vi "filter_param.vi"() -> (0 "shift 0.1":i32, 1 "shift 0.5":i32, 2 "Coeffs Fs=0.1":fxp<+/-,18,18>[](array[numeric]), 3 "Coeffs Fs=0.5":fxp<+/-,18,18>[](array[numeric]))   [LabVIEW 2013]
panel:
  out "sum 0.1":i32
  out "sum 0.5":i32
  out "Waveform Graph":i32[][](graph)
  out "subarray":string[](array[string])
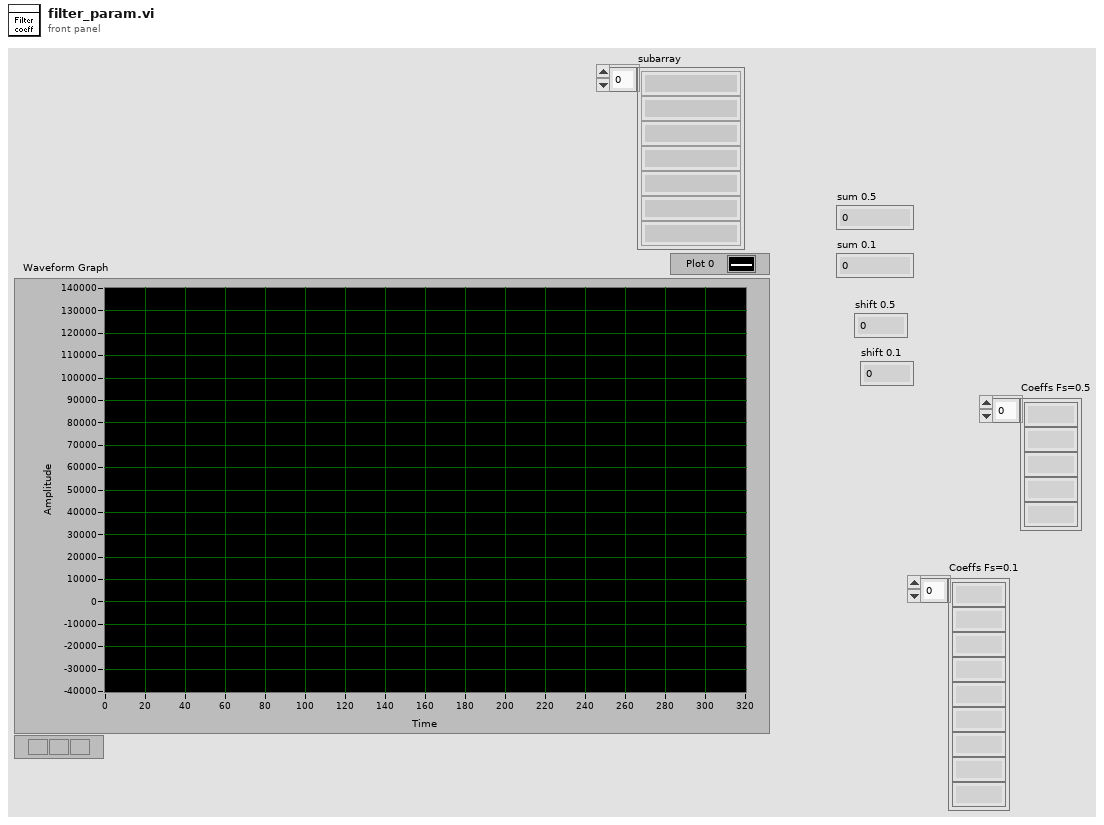
[diagram p1: front panel]
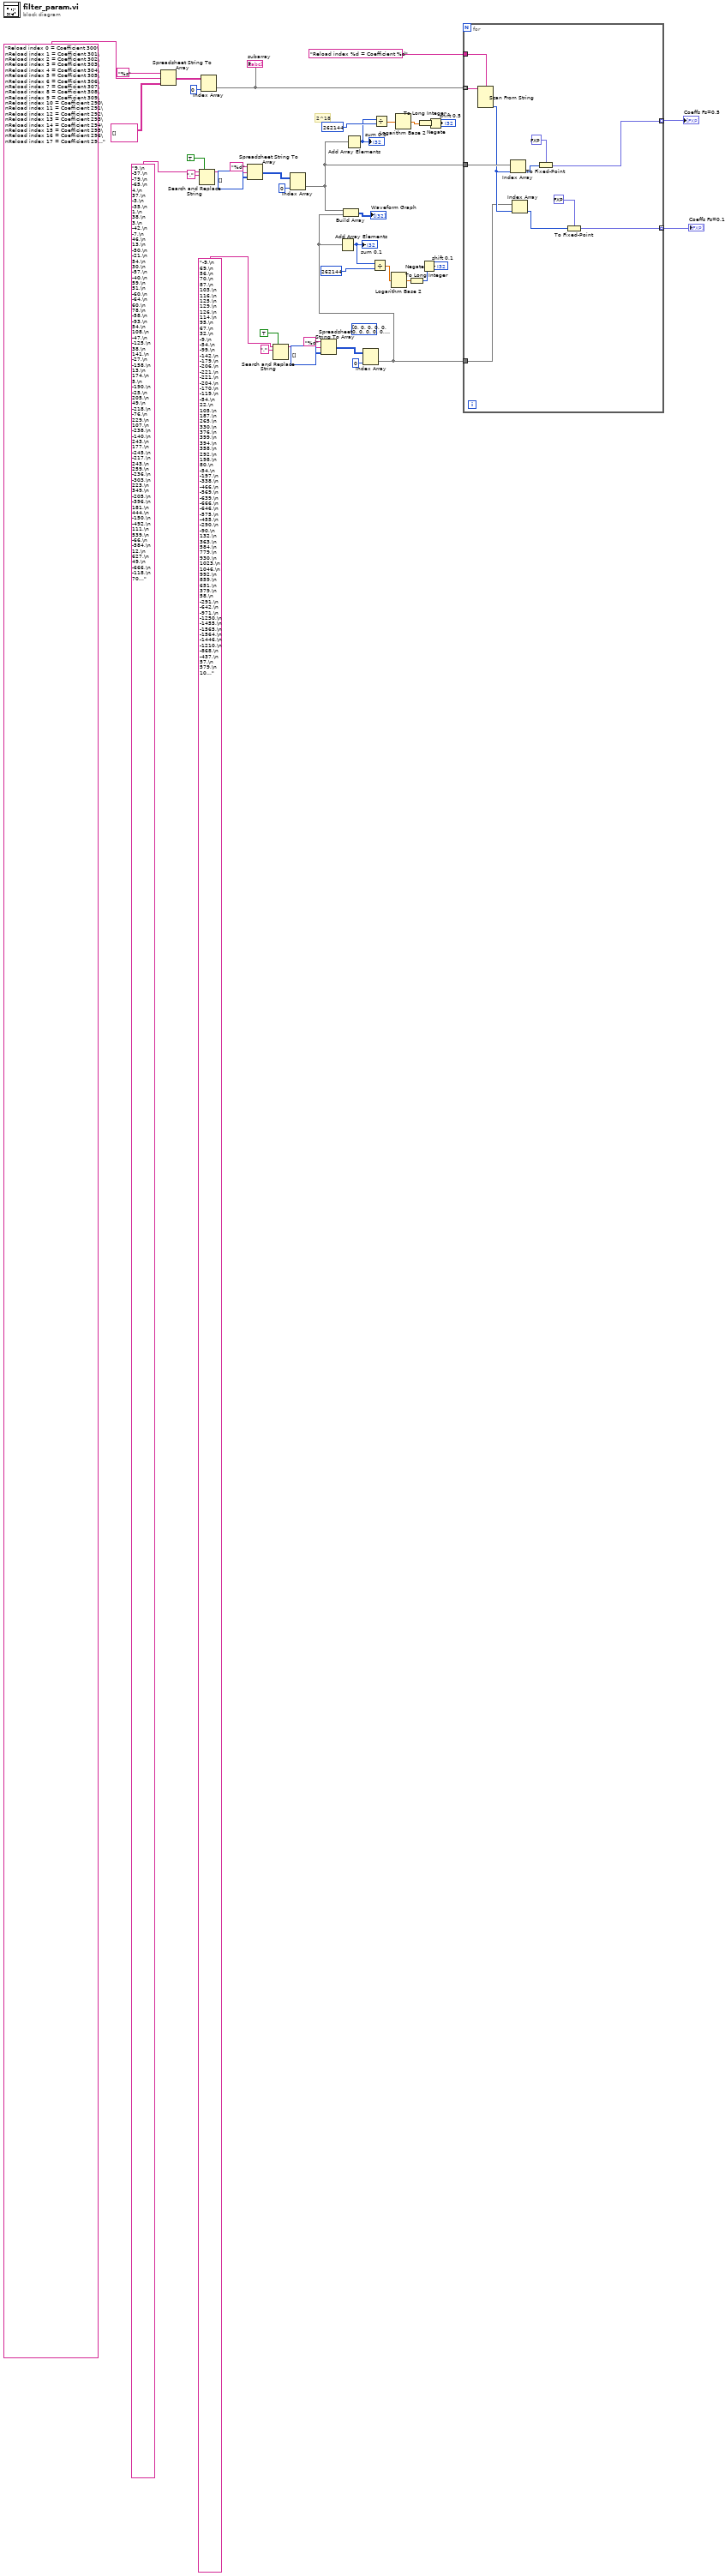
[diagram p0: block diagram]
diagram:
  (unwired) i32[] [0, 0, 0, 0, 0, 0, 0, 0, 0, 0, 0, 0, 0, 0, 0, 0, 0, 0, 0, 0, 0, 0, 0, 0, 0, 0, 0, 0, 0, 0, 0, 0, 0, 0, 0, 0, 0, 0, 0, 0, 0, 0, 0, 0, 0, 0, 0, 0, 0, 0, 0, 0, 0, 0, 0, 0, 0, 0, 0, 0, 0, 0, 0, 0, 0, 0, 0, 0, 0, 0, 0, 0, 0, 0, 0, 0, 0, 0, 0, 0, 0, 0, 0, 0, 0, 0, 0, 0, 0, 0, 0, 0, 0, 0, 0, 0, 0, 0, 0, 0, 0, 0, 0, 0, 0, 0, 0, 0, 0, 0, 0, 0, 0, 0, 0, 0, 0, 0, 0, 0, 0, 0, 0, 0, 0, 0, 0, 0, 0, 0, 0, -22, -91, -234, -449, -668, -741, -465, 327, 1628, 3128, 4186, 3968, 1771, -2547, -8192, -13332, -15398, -11800, -870, 17293, 40433, 64437, 84313, 95575, 95575, 84313, 64437, 40433, 17293, -870, -11800, -15398, -13332, -8192, -2547, 1771, 3968, 4186, 3128, 1628, 327, -465, -741, -668, -449, -234, -91, -22, 0, 0, 0, 0, 0, 0, 0, 0, 0, 0, 0, 0, 0, 0, 0, 0, 0, 0, 0, 0, 0, 0, 0, 0, 0, 0, 0, 0, 0, 0, 0, 0, 0, 0, 0, 0, 0, 0, 0, 0, 0, 0, 0, 0, 0, 0, 0, 0, 0, 0, 0, 0, 0, 0, 0, 0, 0, 0, 0, 0, 0, 0, 0, 0, 0, 0, 0, 0, 0, 0, 0, 0, 0, 0, 0, 0, 0, 0, 0, 0, 0, 0, 0, 0, 0, 0, 0, 0, 0, 0, 0, 0, 0, 0, 0, 0, 0, 0, 0, 0, 0, 0, 0, 0, 0, 0, 0, 0, 0, 0, 0, 0, 0, 0, 0, 0, 0, 0, 0, 0, 0, 0, 0, 0, 0, 0, 0, 0, 0, 0, 0] ("output array")
  # "2^18"
  n1 = Spreadsheet String To Array(format string="%s", spreadsheet string="Reload index 0 = Coefficient 300\nReload index 1 = Coefficient 301\nReload index 2 = Coefficient 302\nReload index 3 = Coefficient 303\nReload index 4 = Coefficient 304\nReload index 5 = Coefficient 305\nReload index 6 = Coefficient 306\nReload index 7 = Coefficient 307\nReload index 8 = Coefficient 308\nReload index 9 = Coefficient 309\nReload index 10 = Coefficient 290\nReload index 11 = Coefficient 291\nReload index 12 = Coefficient 292\nReload index 13 = Coefficient 293\nReload index 14 = Coefficient 294\nReload index 15 = Coefficient 295\nReload index 16 = Coefficient 296\nReload index 17 = Coefficient 297\nReload index 18 = Coefficient 298\nReload index 19 = Coefficient 299\nReload index 20 = Coefficient 280\nReload index 21 = Coefficient 281\nReload index 22 = Coefficient 282\nReload index 23 = Coefficient 283\nReload index 24 = Coefficient 284\nReload index 25 = Coefficient 285\nReload index 26 = Coefficient 286\nReload index 27 = Coefficient 287\nReload index 28 = Coefficient 288\nReload index 29 = Coefficient 289\nReload index 30 = Coefficient 270\nReload index 31 = Coefficient 271\nReload index 32 = Coefficient 272\nReload index 33 = Coefficient 273\nReload index 34 = Coefficient 274\nReload index 35 = Coefficient 275\nReload index 36 = Coefficient 276\nReload index 37 = Coefficient 277\nReload index 38 = Coefficient 278\nReload index 39 = Coefficient 279\nReload index 40 = Coefficient 260\nReload index 41 = Coefficient 261\nReload index 42 = Coefficient 262\nReload index 43 = Coefficient 263\nReload index 44 = Coefficient 264\nReload index 45 = Coefficient 265\nReload index 46 = Coefficient 266\nReload index 47 = Coefficient 267\nReload index 48 = Coefficient 268\nReload index 49 = Coefficient 269\nReload index 50 = Coefficient 250\nReload index 51 = Coefficient 251\nReload index 52 = Coefficient 252\nReload index 53 = Coefficient 253\nReload index 54 = Coefficient 254\nReload index 55 = Coefficient 255\nReload index 56 = Coefficient 256\nReload index 57 = Coefficient 257\nReload index 58 = Coefficient 258\nReload index 59 = Coefficient 259\nReload index 60 = Coefficient 240\nReload index 61 = Coefficient 241\nReload index 62 = Coefficient 242\nReload index 63 = Coefficient 243\nReload index 64 = Coefficient 244\nReload index 65 = Coefficient 245\nReload index 66 = Coefficient 246\nReload index 67 = Coefficient 247\nReload index 68 = Coefficient 248\nReload index 69 = Coefficient 249\nReload index 70 = Coefficient 230\nReload index 71 = Coefficient 231\nReload index 72 = Coefficient 232\nReload index 73 = Coefficient 233\nReload index 74 = Coefficient 234\nReload index 75 = Coefficient 235\nReload index 76 = Coefficient 236\nReload index 77 = Coefficient 237\nReload index 78 = Coefficient 238\nReload index 79 = Coefficient 239\nReload index 80 = Coefficient 220\nReload index 81 = Coefficient 221\nReload index 82 = Coefficient 222\nReload index 83 = Coefficient 223\nReload index 84 = Coefficient 224\nReload index 85 = Coefficient 225\nReload index 86 = Coefficient 226\nReload index 87 = Coefficient 227\nReload index 88 = Coefficient 228\nReload index 89 = Coefficient 229\nReload index 90 = Coefficient 210\nReload index 91 = Coefficient 211\nReload index 92 = Coefficient 212\nReload index 93 = Coefficient 213\nReload index 94 = Coefficient 214\nReload index 95 = Coefficient 215\nReload index 96 = Coefficient 216\nReload index 97 = Coefficient 217\nReload index 98 = Coefficient 218\nReload index 99 = Coefficient 219\nReload index 100 = Coefficient 200\nReload index 101 = Coefficient 201\nReload index 102 = Coefficient 202\nReload index 103 = Coefficient 203\nReload index 104 = Coefficient 204\nReload index 105 = Coefficient 205\nReload index 106 = Coefficient 206\nReload index 107 = Coefficient 207\nReload index 108 = Coefficient 208\nReload index 109 = Coefficient 209\nReload index 110 = Coefficient 190\nReload index 111 = Coefficient 191\nReload index 112 = Coefficient 192\nReload index 113 = Coefficient 193\nReload index 114 = Coefficient 194\nReload index 115 = Coefficient 195\nReload index 116 = Coefficient 196\nReload index 117 = Coefficient 197\nReload index 118 = Coefficient 198\nReload index 119 = Coefficient 199\nReload index 120 = Coefficient 180\nReload index 121 = Coefficient 181\nReload index 122 = Coefficient 182\nReload index 123 = Coefficient 183\nReload index 124 = Coefficient 184\nReload index 125 = Coefficient 185\nReload index 126 = Coefficient 186\nReload index 127 = Coefficient 187\nReload index 128 = Coefficient 188\nReload index 129 = Coefficient 189\nReload index 130 = Coefficient 170\nReload index 131 = Coefficient 171\nReload index 132 = Coefficient 172\nReload index 133 = Coefficient 173\nReload index 134 = Coefficient 174\nReload index 135 = Coefficient 175\nReload index 136 = Coefficient 176\nReload index 137 = Coefficient 177\nReload index 138 = Coefficient 178\nReload index 139 = Coefficient 179\nReload index 140 = Coefficient 160\nReload index 141 = Coefficient 161\nReload index 142 = Coefficient 162\nReload index 143 = Coefficient 163\nReload index 144 = Coefficient 164\nReload index 145 = Coefficient 165\nReload index 146 = Coefficient 166\nReload index 147 = Coefficient 167\nReload index 148 = Coefficient 168\nReload index 149 = Coefficient 169\nReload index 150 = Coefficient 150\nReload index 151 = Coefficient 151\nReload index 152 = Coefficient 152\nReload index 153 = Coefficient 153\nReload index 154 = Coefficient 154\nReload index 155 = Coefficient 155\nReload index 156 = Coefficient 156\nReload index 157 = Coefficient 157\nReload index 158 = Coefficient 158\nReload index 159 = Coefficient 159\nReload index 160 = Coefficient 140\nReload index 161 = Coefficient 141\nReload index 162 = Coefficient 142\nReload index 163 = Coefficient 143\nReload index 164 = Coefficient 144\nReload index 165 = Coefficient 145\nReload index 166 = Coefficient 146\nReload index 167 = Coefficient 147\nReload index 168 = Coefficient 148\nReload index 169 = Coefficient 149\nReload index 170 = Coefficient 130\nReload index 171 = Coefficient 131\nReload index 172 = Coefficient 132\nReload index 173 = Coefficient 133\nReload index 174 = Coefficient 134\nReload index 175 = Coefficient 135\nReload index 176 = Coefficient 136\nReload index 177 = Coefficient 137\nReload index 178 = Coefficient 138\nReload index 179 = Coefficient 139\nReload index 180 = Coefficient 120\nReload index 181 = Coefficient 121\nReload index 182 = Coefficient 122\nReload index 183 = Coefficient 123\nReload index 184 = Coefficient 124\nReload index 185 = Coefficient 125\nReload index 186 = Coefficient 126\nReload index 187 = Coefficient 127\nReload index 188 = Coefficient 128\nReload index 189 = Coefficient 129\nReload index 190 = Coefficient 110\nReload index 191 = Coefficient 111\nReload index 192 = Coefficient 112\nReload index 193 = Coefficient 113\nReload index 194 = Coefficient 114\nReload index 195 = Coefficient 115\nReload index 196 = Coefficient 116\nReload index 197 = Coefficient 117\nReload index 198 = Coefficient 118\nReload index 199 = Coefficient 119\nReload index 200 = Coefficient 100\nReload index 201 = Coefficient 101\nReload index 202 = Coefficient 102\nReload index 203 = Coefficient 103\nReload index 204 = Coefficient 104\nReload index 205 = Coefficient 105\nReload index 206 = Coefficient 106\nReload index 207 = Coefficient 107\nReload index 208 = Coefficient 108\nReload index 209 = Coefficient 109\nReload index 210 = Coefficient 90\nReload index 211 = Coefficient 91\nReload index 212 = Coefficient 92\nReload index 213 = Coefficient 93\nReload index 214 = Coefficient 94\nReload index 215 = Coefficient 95\nReload index 216 = Coefficient 96\nReload index 217 = Coefficient 97\nReload index 218 = Coefficient 98\nReload index 219 = Coefficient 99\nReload index 220 = Coefficient 80\nReload index 221 = Coefficient 81\nReload index 222 = Coefficient 82\nReload index 223 = Coefficient 83\nReload index 224 = Coefficient 84\nReload index 225 = Coefficient 85\nReload index 226 = Coefficient 86\nReload index 227 = Coefficient 87\nReload index 228 = Coefficient 88\nReload index 229 = Coefficient 89\nReload index 230 = Coefficient 70\nReload index 231 = Coefficient 71\nReload index 232 = Coefficient 72\nReload index 233 = Coefficient 73\nReload index 234 = Coefficient 74\nReload index 235 = Coefficient 75\nReload index 236 = Coefficient 76\nReload index 237 = Coefficient 77\nReload index 238 = Coefficient 78\nReload index 239 = Coefficient 79\nReload index 240 = Coefficient 60\nReload index 241 = Coefficient 61\nReload index 242 = Coefficient 62\nReload index 243 = Coefficient 63\nReload index 244 = Coefficient 64\nReload index 245 = Coefficient 65\nReload index 246 = Coefficient 66\nReload index 247 = Coefficient 67\nReload index 248 = Coefficient 68\nReload index 249 = Coefficient 69\nReload index 250 = Coefficient 50\nReload index 251 = Coefficient 51\nReload index 252 = Coefficient 52\nReload index 253 = Coefficient 53\nReload index 254 = Coefficient 54\nReload index 255 = Coefficient 55\nReload index 256 = Coefficient 56\nReload index 257 = Coefficient 57\nReload index 258 = Coefficient 58\nReload index 259 = Coefficient 59\nReload index 260 = Coefficient 40\nReload index 261 = Coefficient 41\nReload index 262 = Coefficient 42\nReload index 263 = Coefficient 43\nReload index 264 = Coefficient 44\nReload index 265 = Coefficient 45\nReload index 266 = Coefficient 46\nReload index 267 = Coefficient 47\nReload index 268 = Coefficient 48\nReload index 269 = Coefficient 49\nReload index 270 = Coefficient 30\nReload index 271 = Coefficient 31\nReload index 272 = Coefficient 32\nReload index 273 = Coefficient 33\nReload index 274 = Coefficient 34\nReload index 275 = Coefficient 35\nReload index 276 = Coefficient 36\nReload index 277 = Coefficient 37\nReload index 278 = Coefficient 38\nReload index 279 = Coefficient 39\nReload index 280 = Coefficient 20\nReload index 281 = Coefficient 21\nReload index 282 = Coefficient 22\nReload index 283 = Coefficient 23\nReload index 284 = Coefficient 24\nReload index 285 = Coefficient 25\nReload index 286 = Coefficient 26\nReload index 287 = Coefficient 27\nReload index 288 = Coefficient 28\nReload index 289 = Coefficient 29\nReload index 290 = Coefficient 10\nReload index 291 = Coefficient 11\nReload index 292 = Coefficient 12\nReload index 293 = Coefficient 13\nReload index 294 = Coefficient 14\nReload index 295 = Coefficient 15\nReload index 296 = Coefficient 16\nReload index 297 = Coefficient 17\nReload index 298 = Coefficient 18\nReload index 299 = Coefficient 19\nReload index 300 = Coefficient 0\nReload index 301 = Coefficient 1\nReload index 302 = Coefficient 2\nReload index 303 = Coefficient 3\nReload index 304 = Coefficient 4\nReload index 305 = Coefficient 5\nReload index 306 = Coefficient 6\nReload index 307 = Coefficient 7\nReload index 308 = Coefficient 8\nReload index 309 = Coefficient 9", array type (2D Dbl)=string[][] []) -> (array=w20:string[][])  [unwired: 1 in]
  n2 = Search and Replace String(replace all?=TRUE ("replace all? (F)"), input string="9,\n   -37,\n   -79,\n   -65,\n     4,\n    37,\n    -3,\n   -35,\n     1,\n    38,\n     3,\n   -42,\n    -7,\n    46,\n    13,\n   -50,\n   -21,\n    54,\n    30,\n   -57,\n   -40,\n    59,\n    51,\n   -60,\n   -64,\n    60,\n    78,\n   -58,\n   -93,\n    54,\n   108,\n   -47,\n  -125,\n    38,\n   141,\n   -27,\n  -158,\n    13,\n   174,\n     5,\n  -190,\n   -25,\n   205,\n    49,\n  -218,\n   -76,\n   229,\n   107,\n  -238,\n  -140,\n   243,\n   177,\n  -245,\n  -217,\n   243,\n   259,\n  -236,\n  -303,\n   223,\n   349,\n  -205,\n  -396,\n   181,\n   444,\n  -150,\n  -492,\n   111,\n   539,\n   -66,\n  -584,\n    12,\n   627,\n    49,\n  -666,\n  -118,\n   700,\n   195,\n  -729,\n  -281,\n   751,\n   373,\n  -765,\n  -473,\n   769,\n   580,\n  -763,\n  -693,\n   746,\n   812,\n  -715,\n  -935,\n   671,\n  1061,\n  -611,\n -1189,\n   535,\n  1319,\n  -442,\n -1447,\n   330,\n  1574,\n  -199,\n -1696,\n    47,\n  1813,\n   126,\n -1921,\n  -320,\n  2019,\n   538,\n -2104,\n  -779,\n  2174,\n  1044,\n -2225,\n -1334,\n  2256,\n  1651,\n -2261,\n -1994,\n  2239,\n  2366,\n -2183,\n -2768,\n  2090,\n  3203,\n -1954,\n -3674,\n  1767,\n  4185,\n -1520,\n -4744,\n  1202,\n  5359,\n  -795,\n -6044,\n   278,\n  6819,\n   384,\n -7715,\n -1242,\n  8781,\n  2385,\n-10100,\n -3964,\n 11816,\n  6282,\n-14214,\n-10018,\n 17920,\n 17062,\n-24561,\n-34982,\n 38856,\n130773,\n130773,\n 38856,\n-34982,\n-24561,\n 17062,\n 17920,\n-10018,\n-14214,\n  6282,\n 11816,\n -3964,\n-10100,\n  2385,\n  8781,\n -1242,\n -7715,\n   384,\n  6819,\n   278,\n -6044,\n  -795,\n  5359,\n  1202,\n -4744,\n -1520,\n  4185,\n  1767,\n -3674,\n -1954,\n  3203,\n  2090,\n -2768,\n -2183,\n  2366,\n  2239,\n -1994,\n -2261,\n  1651,\n  2256,\n -1334,\n -2225,\n  1044,\n  2174,\n  -779,\n -2104,\n   538,\n  2019,\n  -320,\n -1921,\n   126,\n  1813,\n    47,\n -1696,\n  -199,\n  1574,\n   330,\n -1447,\n  -442,\n  1319,\n   535,\n -1189,\n  -611,\n  1061,\n   671,\n  -935,\n  -715,\n   812,\n   746,\n  -693,\n  -763,\n   580,\n   769,\n  -473,\n  -765,\n   373,\n   751,\n  -281,\n  -729,\n   195,\n   700,\n  -118,\n  -666,\n    49,\n   627,\n    12,\n  -584,\n   -66,\n   539,\n   111,\n  -492,\n  -150,\n   444,\n   181,\n  -396,\n  -205,\n   349,\n   223,\n  -303,\n  -236,\n   259,\n   243,\n  -217,\n  -245,\n   177,\n   243,\n  -140,\n  -238,\n   107,\n   229,\n   -76,\n  -218,\n    49,\n   205,\n   -25,\n  -190,\n     5,\n   174,\n    13,\n  -158,\n   -27,\n   141,\n    38,\n  -125,\n   -47,\n   108,\n    54,\n   -93,\n   -58,\n    78,\n    60,\n   -64,\n   -60,\n    51,\n    59,\n   -40,\n   -57,\n    30,\n    54,\n   -21,\n   -50,\n    13,\n    46,\n    -7,\n   -42,\n     3,\n    38,\n     1,\n   -35,\n    -3,\n    37,\n     4,\n   -65,\n   -79,\n   -37,\n     9", search string=",") -> (result string=w37:string)  [unwired: 5 in, 3 out]
  n3 = Index Array(array=w20, index (col)=0 ("disabled index (col)")) -> (element=w19:string[])  [unwired: 1 in]
  "subarray" <- w19
  n4 = Spreadsheet String To Array(format string="%d", spreadsheet string=w37, array type (2D Dbl)=i32[][] []) -> (array=w34:i32[][])  [unwired: 1 in]
  n5 = Search and Replace String(replace all?=TRUE ("replace all? (F)"), input string="-9,\n    69,\n    56,\n    70,\n    87,\n   103,\n   116,\n   125,\n   129,\n   126,\n   114,\n    95,\n    67,\n    32,\n    -9,\n   -54,\n   -99,\n  -142,\n  -179,\n  -206,\n  -221,\n  -221,\n  -204,\n  -170,\n  -119,\n   -54,\n    22,\n   105,\n   187,\n   265,\n   330,\n   376,\n   399,\n   394,\n   358,\n   292,\n   198,\n    80,\n   -54,\n  -197,\n  -338,\n  -466,\n  -569,\n  -639,\n  -666,\n  -646,\n  -575,\n  -455,\n  -290,\n   -90,\n   132,\n   363,\n   584,\n   779,\n   930,\n  1023,\n  1046,\n   992,\n   859,\n   651,\n   379,\n    58,\n  -291,\n  -642,\n  -971,\n -1250,\n -1455,\n -1565,\n -1564,\n -1446,\n -1210,\n  -868,\n  -437,\n    57,\n   579,\n  1093,\n  1559,\n  1939,\n  2198,\n  2308,\n  2252,\n  2024,\n  1628,\n  1084,\n   423,\n  -312,\n -1071,\n -1798,\n -2436,\n -2931,\n -3238,\n -3321,\n -3159,\n -2749,\n -2106,\n -1264,\n  -274,\n   800,\n  1882,\n  2891,\n  3748,\n  4376,\n  4716,\n  4723,\n  4374,\n  3673,\n  2650,\n  1361,\n  -117,\n -1684,\n -3228,\n -4634,\n -5785,\n -6579,\n -6931,\n -6784,\n -6115,\n -4935,\n -3296,\n -1287,\n   970,\n  3326,\n  5613,\n  7654,\n  9279,\n 10334,\n 10691,\n 10266,\n  9021,\n  6974,\n  4203,\n   841,\n -2921,\n -6850,\n-10676,\n-14110,\n-16859,\n-18641,\n-19208,\n-18358,\n-15950,\n-11918,\n -6277,\n   871,\n  9344,\n 18880,\n 29150,\n 39774,\n 50337,\n 60410,\n 69573,\n 77436,\n 83657,\n 87964,\n 90166,\n 90166,\n 87964,\n 83657,\n 77436,\n 69573,\n 60410,\n 50337,\n 39774,\n 29150,\n 18880,\n  9344,\n   871,\n -6277,\n-11918,\n-15950,\n-18358,\n-19208,\n-18641,\n-16859,\n-14110,\n-10676,\n -6850,\n -2921,\n   841,\n  4203,\n  6974,\n  9021,\n 10266,\n 10691,\n 10334,\n  9279,\n  7654,\n  5613,\n  3326,\n   970,\n -1287,\n -3296,\n -4935,\n -6115,\n -6784,\n -6931,\n -6579,\n -5785,\n -4634,\n -3228,\n -1684,\n  -117,\n  1361,\n  2650,\n  3673,\n  4374,\n  4723,\n  4716,\n  4376,\n  3748,\n  2891,\n  1882,\n   800,\n  -274,\n -1264,\n -2106,\n -2749,\n -3159,\n -3321,\n -3238,\n -2931,\n -2436,\n -1798,\n -1071,\n  -312,\n   423,\n  1084,\n  1628,\n  2024,\n  2252,\n  2308,\n  2198,\n  1939,\n  1559,\n  1093,\n   579,\n    57,\n  -437,\n  -868,\n -1210,\n -1446,\n -1564,\n -1565,\n -1455,\n -1250,\n  -971,\n  -642,\n  -291,\n    58,\n   379,\n   651,\n   859,\n   992,\n  1046,\n  1023,\n   930,\n   779,\n   584,\n   363,\n   132,\n   -90,\n  -290,\n  -455,\n  -575,\n  -646,\n  -666,\n  -639,\n  -569,\n  -466,\n  -338,\n  -197,\n   -54,\n    80,\n   198,\n   292,\n   358,\n   394,\n   399,\n   376,\n   330,\n   265,\n   187,\n   105,\n    22,\n   -54,\n  -119,\n  -170,\n  -204,\n  -221,\n  -221,\n  -206,\n  -179,\n  -142,\n   -99,\n   -54,\n    -9,\n    32,\n    67,\n    95,\n   114,\n   126,\n   129,\n   125,\n   116,\n   103,\n    87,\n    70,\n    56,\n    69,\n    -9", search string=",") -> (result string=w28:string)  [unwired: 5 in, 3 out]
  n6 = Index Array(array=w34, index (col)=0 ("disabled index (col)")) -> (element=w14:i32[])  [unwired: 1 in]
  n7 = Spreadsheet String To Array(format string="%d", spreadsheet string=w28, array type (2D Dbl)=i32[][] []) -> (array=w31:i32[][])  [unwired: 1 in]
  n8 = Add Array Elements(numeric array=w14) -> (sum=w11:i32)
  "sum 0.5" <- w11
  n9 = Index Array(array=w31, index (col)=0 ("disabled index (col)")) -> (element=w13:i32[])  [unwired: 1 in]
  n10 = Add Array Elements(numeric array=w13) -> (sum=w9:i32)
  "sum 0.1" <- w9
  n11 = Build Array(w14, w13) -> (→"Waveform Graph":i32[][])
  n12 = Divide(x=w9, y=262144 ("sum 0.5")) -> (x/y=w7:dbl)
  n13 = Divide(x=w11, y=262144 ("sum 0.5")) -> (x/y=w4:dbl)
  n14 = Logarithm Base 2(1:w7) -> (0:w6:dbl)
  n15 = Logarithm Base 2(1:w4) -> (0:w3:dbl)
  n16 = To Long Integer(number=w6) -> (32bit integer=w5:i32)
  n17 = To Long Integer(number=w3) -> (32bit integer=w10:i32)
  n18 = Negate(x=w5) -> (-x=→"shift 0.1":i32)
  n19 = Negate(x=w10) -> (-x=→"shift 0.5":i32)
  n20 = for {
    tunnel: w14 -> [w47]
    tunnel: w13 -> [w41]
    tunnel: w19 -> [w50] mode=indexing
    tunnel: "Reload index %d = Coefficient %d" -> [w49]
    tunnel: [w45] -> w17 mode=indexing
    tunnel: [w42] -> w16 mode=indexing
    n21 = Scan From String(format string=w49, input string=w50) -> (output 2=w44:i32)  [unwired: 5 in, 3 out]
    n22 = Index Array(array=w47, index=w44) -> (element=w46:i32)
    n23 = Index Array(array=w41, index=w44) -> (element=w43:i32)
    n24 = To Fixed-Point(fixed-point type=fxp<+/-,18,18> 0.0 ("s_axis_reload_tdata 2"), number=w46) -> (fixed-point=w45:fxp<+/-,18,18>)
    n25 = To Fixed-Point(fixed-point type=fxp<+/-,18,18> 0.0 ("s_axis_reload_tdata 2"), number=w43) -> (fixed-point=w42:fxp<+/-,18,18>)
  }
  "Coeffs Fs=0.5" <- w17
  "Coeffs Fs=0.1" <- w16
